vi "read-T.vi"(8 "error in (no error)":errorcluster, 11 "temperature reader.lvclass":refnum<class "temperature reader.lvclass">) -> (0 "error out":errorcluster, 2 "Result":dbl[](array[numeric]), 3 "temperature reader.lvclass Out":refnum<class "temperature reader.lvclass">)   [LabVIEW 2018, in "temperature reader.lvclass"]
uses:
  temperature reader.lvclass
  Users/Shared/github/NHMFL_Core/Libraries/Instruments/Instrument Driver/Instrument Driver.lvclass
  resonant_ultrasound_arxiv/maglab ultrasound -- arkady --arxiv/publisher action.ctl
  NHMFL_Core/Libraries/Instruments/Instrument Driver/Instrument Driver.lvclass/Instrument Driver.ctl
  NHMFL_Core/Libraries/Instruments/Instrument Driver/Write Channel names.vi
  NHMFL_Core/Libraries/Instruments/Instrument Driver/Write Channel units.vi
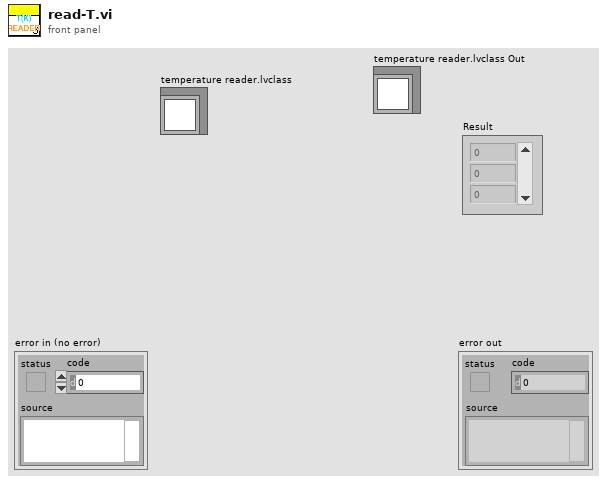
[diagram p1: front panel]
types:
  T1 = typedef "publisher action.ctl" = enum16{"set", "get"}
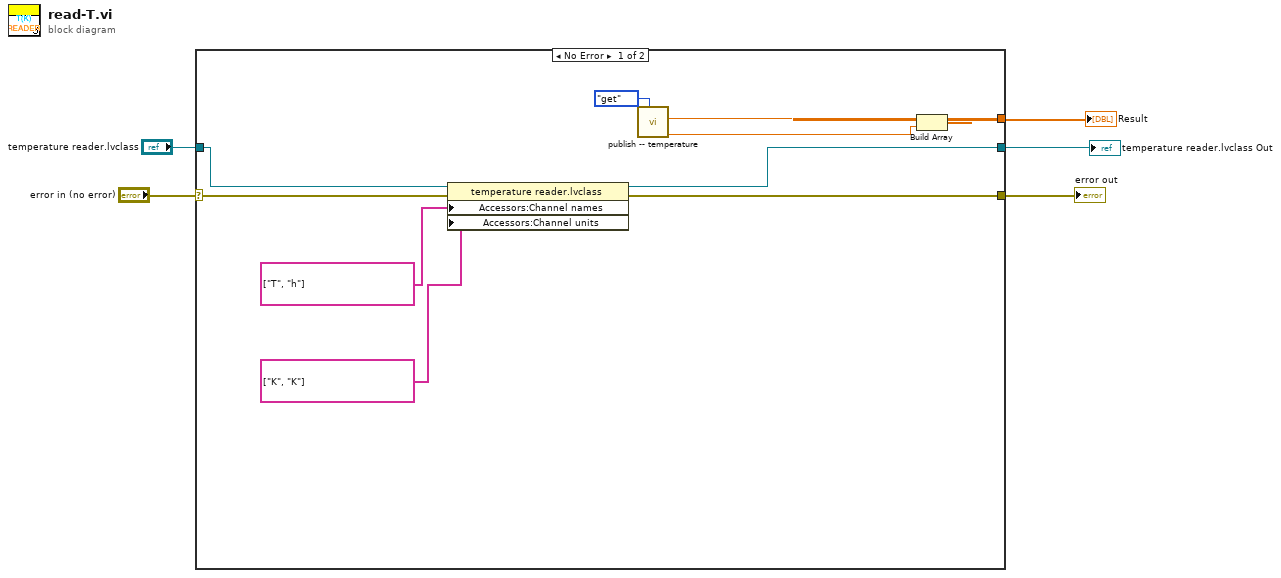
[diagram p0: block diagram]
diagram:
  n1 = case shown="No Error" "error in (no error)" {
    selector: "error in (no error)" -> [w12 w17]
    tunnel: [w11 w17] -> w4
    tunnel: [w13 w16] -> w2
    tunnel: "temperature reader.lvclass" -> [w14 w16]
    tunnel: [w15 _] -> w3
    frame No Error {
      n2 = property class="temperature reader.lvclass"(reference=w14, error in=w12, "Accessors:Channel names"=string[] ["T", "h"] ("Channel names"), "Accessors:Channel units"=string[] ["K", "K"] ("Channel names")) -> (reference out=w13:refnum<class "temperature reader.lvclass">, error out=w11:errorcluster)
      n3 = call "publish -- temperature.vi"("publisher action"=publisher_action."get") -> ("heater OUT"=w6:dbl, "T (K) OUT"=w7:dbl)  [unwired: 9 in]
      n4 = Build Array(w7, w6) -> (w15:dbl[])
    }
    frame Error {
    }
  }
  "error out" <- w4
  "Result" <- w3
  "temperature reader.lvclass Out" <- w2
